vi "Scalar to Variant Array.vi"(2 "error in (no error)":errorcluster, 3 "Scalar Variant":variant) -> (0 "error out":errorcluster, 1 "1-D Array Variant":variant)   [LabVIEW 2017]
uses:
  <userlib>/_OpenG.lib/lvdata/lvdata.llb/Type Descriptor Enumeration__ogtk.ctl
panel:
  # "LVHDF5 Toolkit\nCopyright (c) 2005-2013 by Jason D. Sommerville\nCopyright (c) 2014 by UPVI, LLC.\n\nThis use and distribution of this file is governed by the terms found in \nLICENSE.txt distributed with this toolkit and installed at\n <user.lib>\\_lvhdf5\\LICENSE.txt"
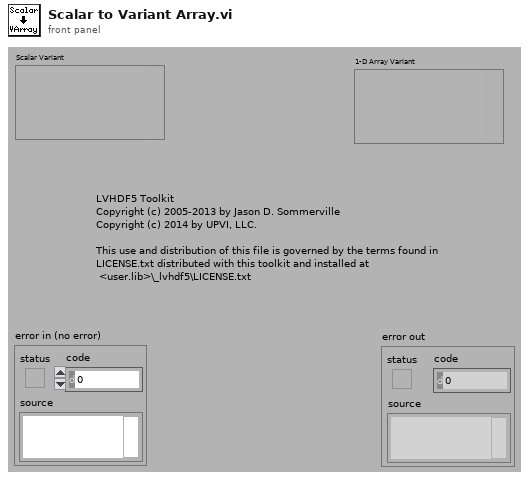
[diagram p1: front panel]
types:
  T1 = typedef "Type Descriptor Enumeration__ogtk.ctl" = enum8{"<Null>", "I8", "I16", "I32", "I64", "U8", "U16", "U32", "U64", "SGL", "DBL", "EXT", "CSG", "CDB", "CXT", "0x0F", "0x10", "0x11", "0x12", "0x13", "0x14", "Enum U8", "Enum U16", "Enum U32", "Enum U64", "SGL PQ", "DBL PQ", "EXT PQ", "CSG PQ", "CDB PQ", "CXT PQ", "0x1F", "0x20", "Boolean", "0x22", "0x23", "0x24", "0x25", "0x26", "0x27", "0x28", "0x29", "0x2A", "0x2B", "0x2C", "0x2D", "0x2E", "0x2F", "String", "0x31", "Path", "Pict", "0x34", "0x35", "0x36", "DAQ", "0x38", "0x39", "0x3A", "0x3B", "0x3C", "0x3D", "0x3E", "0x3F", "Array", "0x41", "0x42", "0x43", "0x44", "0x45", "0x46", "0x47", "0x48", "0x49", "0x4A", "0x4B", "0x4C", "0x4D", "0x4E", "0x4F", "Cluster", "0x51", "0x52", "Variant", "Waveform", "0x55", "0x56", "0x57", "0x58", "0x59", "0x5A", "0x5B", "0x5C", "0x5D", "0x5E", "0x5F", "0x60", "0x61", "0x62", "0x63", "0x64", "0x65", "0x66", "0x67", "0x68", "0x69", "0x6A", "0x6B", "0x6C", "0x6D", "0x6E", "0x6F", "Refnum"}
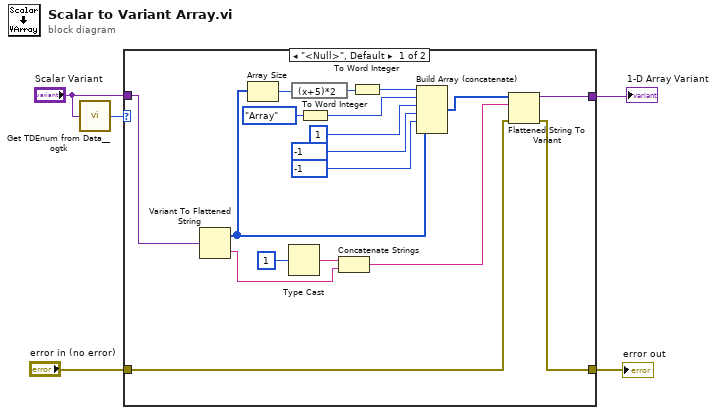
[diagram p0: block diagram]
diagram:
  n1 = call <userlib>:"Get TDEnum from Data__ogtk.vi"("Data"="Scalar Variant") -> ("Type Descriptor Enumeration"=w5:T1)  [unwired: 4 in]
  n2 = case shown="\"<Null>\", Default" w5 {
    tunnel: "Scalar Variant" -> [w23 w25]
    tunnel: "error in (no error)" -> [w8 w24]
    tunnel: [w7 w24] -> w2
    tunnel: [w6 w25] -> w1
    frame "<Null>", Default {
      n3 = Variant To Flattened String(Variant=w23) -> (data string=w11:string, 1:w13:i16[])
      n4 = Array Size(array=w13) -> (size(s)=w20:i32)
      n5 = Type Cast(x=1) -> (*(type *) &x=w12:string)  [unwired: 1 in]
      n6 = expression code="(x+5)*2"(w20) -> (w19:i32)
      n7 = To Word Integer(number=Type_Descriptor_Enumeration__ogtk."Array" ("Type Descriptor Enumeration")) -> (16bit integer=w17:i16)
      n8 = Concatenate Strings(w12, w11) -> (w9:string)
      n9 = To Word Integer(number=w19) -> (16bit integer=w18:i16)
      n10 = Build Array (concatenate)(w18, w17, i16 1, i16 -1, i16 -1, w13) -> (w10:i16[])
      n11 = Flattened String To Variant(4:w8, 6:w9, 7:w10) -> (0:w7:errorcluster, 3:w6:variant)
    }
    frame "Array" {
      # "Already an array"
    }
  }
  "1-D Array Variant" <- w1
  "error out" <- w2
